vi "Write Control RefNums.vi"(8 "error in (no error)":errorcluster, 10 "Control RefNums":T1, 11 "UserInterface in":refnum<class "UserInterface.lvclass">) -> (0 "error out":errorcluster, 3 "UserInterface out":refnum<class "UserInterface.lvclass">)   [LabVIEW 2022 SP3, in "UserInterface.lvlib" / "UserInterface.lvclass"]
uses:
  UserInterface.lvclass
  UserInterface.lvclass/UserInterface.ctl
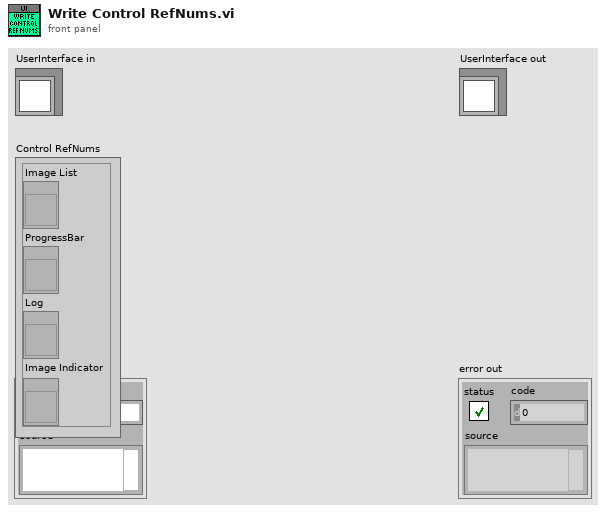
[diagram p1: front panel]
types:
  T1 = cluster{"Image List":refnum<vi>, "ProgressBar":refnum<vi>, "Log":refnum<vi>, "Image Indicator":refnum<vi>}
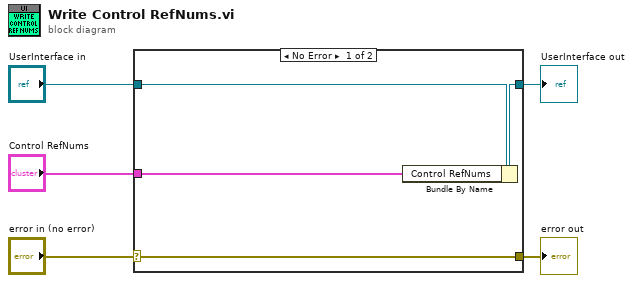
[diagram p0: block diagram]
diagram:
  n1 = case shown="No Error" "error in (no error)" {
    selector: "error in (no error)" -> [w9 w10]
    tunnel: [w9 w10] -> w4
    tunnel: [w7 w11] -> w2
    tunnel: "UserInterface in" -> [w8 w11]
    tunnel: "Control RefNums" -> [w6 _]
    frame No Error {
      n2 = Bundle By Name(cluster=w8, "Control RefNums"=w6) -> (w7:refnum<class "UserInterface.lvclass">)
    }
    frame Error {
    }
  }
  "error out" <- w4
  "UserInterface out" <- w2
